vi "Relay - queue mode.vi"(8 "error in (no error)":errorcluster) -> (0 "error out":errorcluster)   [LabVIEW 2026, in "Tests.lvlib"]
doc: "Integration test. Verifies that a single Log call fans out to every registered appender: registers three queue-mode relay appenders, logs one Info message, and asserts each appender's queue receives exactly one Statement with identical payload. Every gate except fan-out is held open (global threshold at floor, permissive filters, unbounded queues), so a missing element can only be a fan-out defect.\n\nImplements LMBR-T-030 -> SRS-019, SRS-028. Assert-level IDs: Test-ID-Assert-Checklist.md."
uses:
  Tests.lvlib
  src/TypeDefs/Severity.ctl
  <vilib>/addons/_JKI Toolkits/Caraya/classes/Assert/Assert True.vi
  <vilib>/addons/_JKI Toolkits/Caraya/classes/Test/Test.lvclass
  src/Lumberjack.lvlib
  src/Public/Logger.lvclass/Logger.lvclass
  <vilib>/addons/_JKI Toolkits/Caraya/classes/Assert/Assert.lvclass
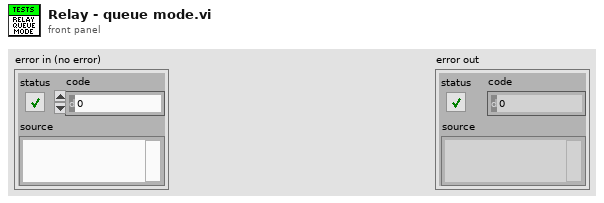
[diagram p1: front panel]
types:
  T1 = typedef "Lumberjack.lvlib/Severity.ctl" = enum16{"OFF", "FATAL", "ERROR", "WARN", "INFO", "DEBUG", "TRACE", "ALL"}
  T2 = typedef "Lumberjack.lvlib/Statement.ctl" = cluster{"timestamp":timestamp, "level":T1, "sourceTag":string, "originVI":string, "message":string}
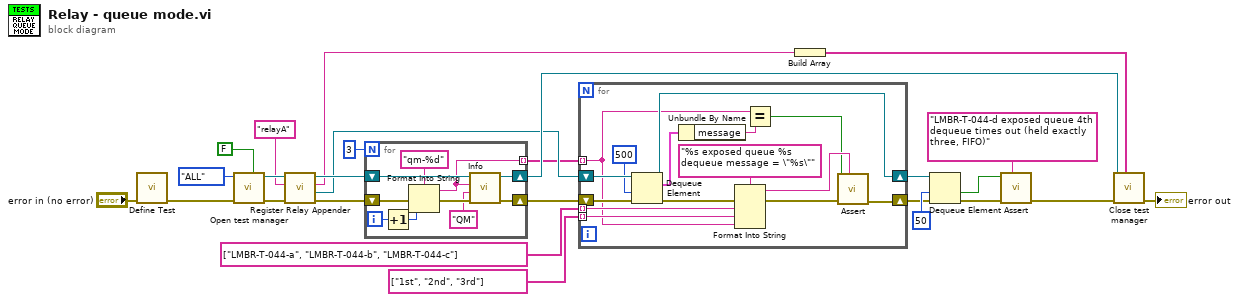
[diagram p0: block diagram]
diagram:
  n1 = call <vilib>:"Define Test.vi"("error in (no error)"="error in (no error)") -> ("error out"=w25:errorcluster)  [unwired: 9 in, 1 out]
  n2 = call "Open test manager.vi"("enableDefaultFile"=FALSE, "error in (no error)"=w25, "globalThreshold"=Severity."ALL") -> ("error out"=w19:errorcluster, "Logger out"=w20:refnum<class "Logger.lvclass">)  [unwired: 7 in]
  n3 = call "Register Relay Appender.vi"("error in (no error)"=w19, "id in"="relayA", "Logger in"=w20) -> ("error out"=w17:errorcluster, "relayQueue"=w16:refnum<queue>, "id out"=w2:string, "Logger out"=w18:refnum<class "Logger.lvclass">)  [unwired: 5 in]
  n4 = for {
    N: 3 -> [_]
    shift-right: [w35] -> w21
    shift-left: w18 -> [w34]
    shift-right: [w36] -> w23
    shift-left: w17 -> [w33]
    tunnel: [w28] -> w7 mode=indexing
    i -> [w29]
    n5 = Increment(x=w29) -> (x+1=w30:i32)
    n6 = Format Into String(format string="qm-%d" ("message"), error in=w33, w30) -> (resulting string=w28:string, error out=w32:errorcluster)  [unwired: 1 in]
    n7 = call "Info.vi"("error in (no error)"=w32, "sourceTag"="QM", "message"=w28, "Logger in"=w34) -> ("error out"=w36:errorcluster, "Logger out"=w35:refnum<class "Logger.lvclass">)  [unwired: 6 in]
  }
  n8 = for {
    shift-right: [w42] -> w4
    shift-left: w23 -> [w51]
    shift-right: [w48] -> w9
    shift-left: w16 -> [w50]
    tunnel: w7 -> [w37] mode=indexing
    tunnel: string[] ["LMBR-T-044-a", "LMBR-T-044-b", "LMBR-T-044-c"] -> [w46] mode=indexing
    tunnel: string[] ["1st", "2nd", "3rd"] -> [w45] mode=indexing
    n9 = Dequeue Element(queue=w50, timeout in ms (-1)=500, error in (no error)=w51) -> (queue out=w48:refnum<queue>, element=w41:T2, error out=w44:errorcluster)  [unwired: 1 out]
    n10 = Unbundle By Name(w41) -> ("message"=w39:string)
    n11 = Format Into String(format string="%s exposed queue %s dequeue message = \"%s\"" ("Label"), error in=w44, w46, w45, w37) -> (resulting string=w40:string, error out=w43:errorcluster)  [unwired: 1 in]
    n12 = Equal?(x=w37, y=w39) -> (x = y?=w38:bool)
    n13 = call-poly <vilib>:"Assert.vi"("Label"=w40, "error in (no error)"=w43, "True?"=w38) -> ("error out"=w42:errorcluster)  [unwired: 7 in, 1 out]
  }
  n14 = Build Array(w2) -> (w1:string[])
  n15 = Dequeue Element(queue=w9, timeout in ms (-1)=50, error in (no error)=w4) -> (timed out?=w8:bool, error out=w10:errorcluster)  [unwired: 2 out]
  n16 = call-poly <vilib>:"Assert.vi"("Label"="LMBR-T-044-d exposed queue 4th dequeue times out (held exactly three, FIFO)", "error in (no error)"=w10, "True?"=w8) -> ("error out"=w15:errorcluster)  [unwired: 7 in, 1 out]
  n17 = call "Close test manager.vi"("queueIDList"=w1, "error in (no error)"=w15, "Logger in"=w21) -> ("error out"=→"error out":errorcluster)  [unwired: 6 in]
